vi "加载类实例.vi"(8 "error in (no error)":errorcluster caption="错误输入（无错误）") -> (0 "error out":errorcluster caption="错误输出", 3 "数组":refnum<class "命令类.lvclass">[](array[class]))   [LabVIEW 2011]
doc: "该模板用于创建子VI。"
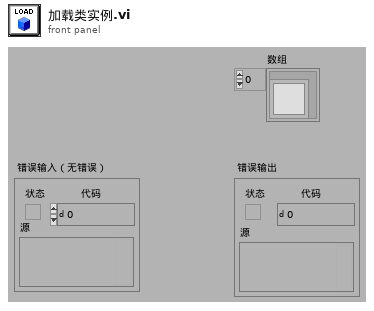
[diagram p1: front panel]
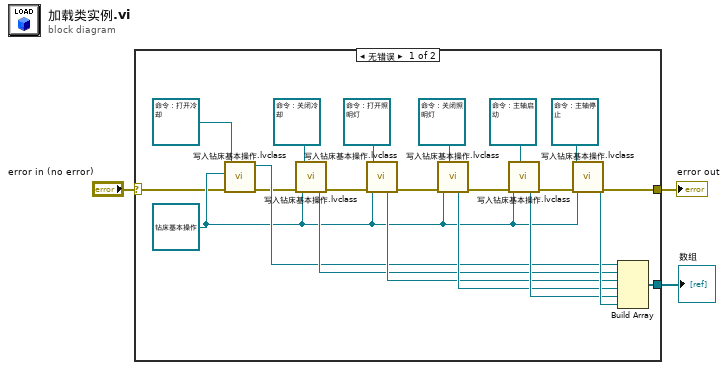
[diagram p0: block diagram]
diagram:
  n1 = case shown="无错误" "error in (no error)" {
    selector: "error in (no error)" -> [w10 w25]
    tunnel: [w4 w25] -> w2
    tunnel: [w11 _] -> w1
    frame No Error {
      w17 = refnum<class "钻床基本操作.lvclass"> refnum ("钻床基本操作.lvclass")
      n2 = call "写入钻床基本操作.lvclass.vi"("error in (no error)"=w10, "钻床基本操作.lvclass"=w17, "命令：打开冷却输入"=refnum<class "命令：打开冷却.lvclass"> refnum ("命令：打开冷却.lvclass")) -> ("error out"=w9:errorcluster, "命令：打开冷却输出"=w19:refnum<class "命令：打开冷却.lvclass">)  [unwired: 7 in]
      n3 = call "写入钻床基本操作.lvclass.vi"("error in (no error)"=w9, "钻床基本操作.lvclass"=w17, "命令：打开冷却输入"=refnum<class "命令：关闭冷却.lvclass"> refnum ("命令：关闭冷却.lvclass")) -> ("error out"=w8:errorcluster, "命令：打开冷却输出"=w20:refnum<class "命令：关闭冷却.lvclass">)  [unwired: 7 in]
      n4 = call "写入钻床基本操作.lvclass.vi"("error in (no error)"=w8, "钻床基本操作.lvclass"=w17, "命令：打开照明灯输入"=refnum<class "命令：打开照明灯.lvclass"> refnum ("命令：打开照明灯.lvclass")) -> ("error out"=w7:errorcluster, "命令：打开照明灯输出"=w21:refnum<class "命令：打开照明灯.lvclass">)  [unwired: 7 in]
      n5 = call "写入钻床基本操作.lvclass.vi"("error in (no error)"=w7, "钻床基本操作.lvclass"=w17, "命令：关闭照明灯输入"=refnum<class "命令：关闭照明灯.lvclass"> refnum ("命令：关闭照明灯.lvclass")) -> ("error out"=w6:errorcluster, "命令：关闭照明灯输出"=w22:refnum<class "命令：关闭照明灯.lvclass">)  [unwired: 7 in]
      n6 = call "写入钻床基本操作.lvclass.vi"("error in (no error)"=w6, "钻床基本操作.lvclass"=w17, "命令：打开冷却输入"=refnum<class "命令：主轴启动.lvclass"> refnum ("命令：主轴启动.lvclass")) -> ("error out"=w5:errorcluster, "命令：打开冷却输出"=w23:refnum<class "命令：主轴启动.lvclass">)  [unwired: 7 in]
      n7 = call "写入钻床基本操作.lvclass.vi"("error in (no error)"=w5, "钻床基本操作.lvclass"=w17, "命令：主轴停止输入"=refnum<class "命令：主轴停止.lvclass"> refnum ("命令：主轴停止.lvclass")) -> ("error out"=w4:errorcluster, "命令：主轴停止输出"=w24:refnum<class "命令：主轴停止.lvclass">)  [unwired: 7 in]
      n8 = Build Array(w19, w20, w21, w22, w23, w24) -> (w11:refnum<class "命令类.lvclass">[])
    }
    frame Error {
    }
  }
  "error out" <- w2
  "数组" <- w1
